vi "Encode String Escape Characters.vi"(1 "unescaped string in":string) -> (0 "escaped string out":string)   [LabVIEW 2010, in "i3-json.lvlib"]
doc: "Percent encodes the supplied string."
uses:
  i3-json.lvlib
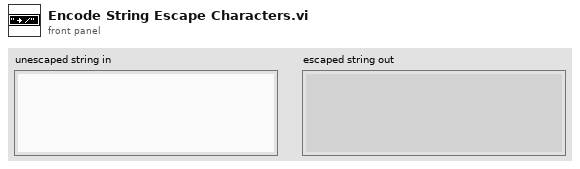
[diagram p1: front panel]
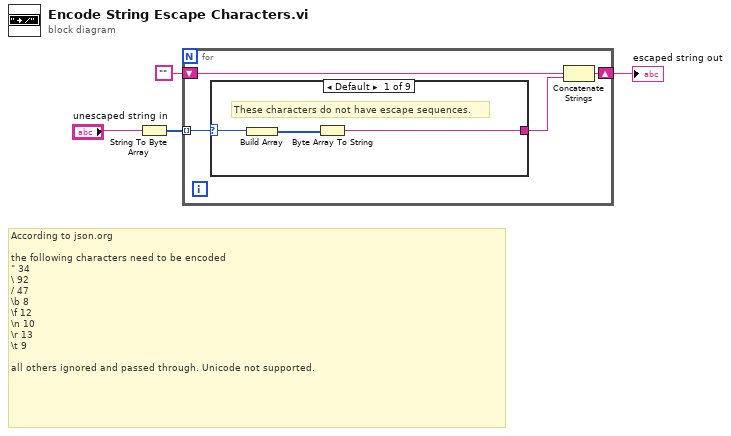
[diagram p0: block diagram]
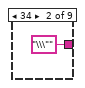
[diagram p2: hidden frame]
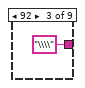
[diagram p3: hidden frame]
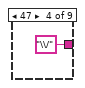
[diagram p4: hidden frame]
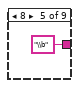
[diagram p5: hidden frame]
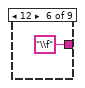
[diagram p6: hidden frame]
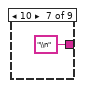
[diagram p7: hidden frame]
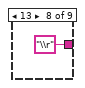
[diagram p8: hidden frame]
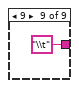
[diagram p9: hidden frame]
diagram:
  # "According to json.org\n\nthe following characters need to be encoded\n\" 34\n\\ 92\n/ 47\n\\b 8\n\\f 12\n\\n 10\n\\r 13\n\\t 9\n\nall others ignored and passed through. Unicode not supported."
  n1 = String To Byte Array(string="unescaped string in") -> (unsigned byte array=w1:u8[])
  n2 = for {
    shift-right: [w5] -> w4
    shift-left: "" -> [w6]
    tunnel: w1 -> [w8] mode=indexing
    n3 = case shown="Default" w8 {
      selector: w8 -> [w11 _ _ _ _ _ _ _ _]
      tunnel: [w9 "\\\"" ("string") "\\\\" ("string") "\\/" ("string") "\\b" ("string") "\\f" ("string") "\\n" ("string") "\\r" ("string") "\\t" ("string")] -> w7
      frame Default {
        # "These characters do not have escape sequences."
        n4 = Build Array(w11) -> (w10:u8[])
        n5 = Byte Array To String(unsigned byte array=w10) -> (string=w9:string)
      }
      frame 34 {
      }
      frame 92 {
      }
      frame 47 {
      }
      frame 8 {
      }
      frame 12 {
      }
      frame 10 {
      }
      frame 13 {
      }
      frame 9 {
      }
    }
    n6 = Concatenate Strings(w6, w7) -> (w5:string)
  }
  "escaped string out" <- w4
